vi "connect to machine.vi"(0 "connection ID":refnum<k5>, 2 "news":string, 5 "error in (no error)":errorcluster) -> (14 "connection ID out":refnum<k5>, 16 "reply":string, 19 "error out":errorcluster)   [LabVIEW 2011]
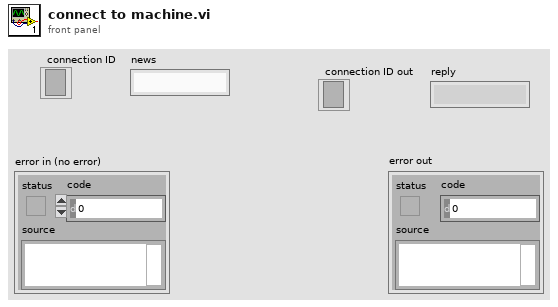
[diagram p1: front panel]
types:
  T1 = enum16{"Standard", "Buffered", "CRLF", "Immediate"}
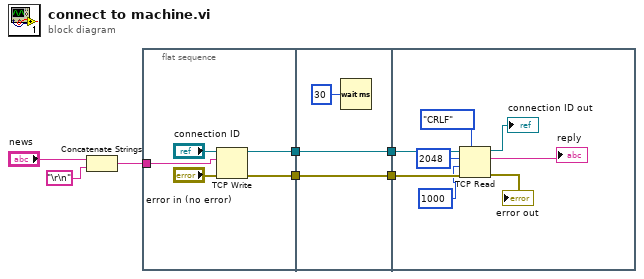
[diagram p0: block diagram]
diagram:
  n1 = Concatenate Strings("news", "\r\n") -> (w6:string)
  n2 = flat-sequence {
    tunnel: w6 -> [w10]
    tunnel: [w9] -> w4
    tunnel: [w8] -> w2
    tunnel: [w14] -> w5
    tunnel: w4 -> [w14]
    tunnel: [w13] -> w3
    tunnel: w2 -> [w13]
    tunnel: w5 -> [w23]
    tunnel: w3 -> [w22]
    frame #0 {
      n3 = TCP Write(connection ID="connection ID", data in=w10, error in (no error)="error in (no error)") -> (connection ID out=w9:refnum<k5>, error out=w8:errorcluster)  [unwired: 1 in, 1 out]
    }
    frame #1 {
      n4 = Wait (ms)(milliseconds to wait=u32 30) -> ()  [unwired: 1 out]
    }
    frame #2 {
      n5 = TCP Read(connection ID=w23, bytes to read=2048, error in (no error)=w22, 7:T1."CRLF" ("mode (standard)"), 9:1000 ("timeout ms (25000)")) -> (connection ID out=→"connection ID out":refnum<k5>, data out=→"reply":string, error out=→"error out":errorcluster)
    }
  }
